vi "multiply value.vi"(6 "label":T1, 8 "error in (no error)":errorcluster, 10 "B":refnum<class "Value.lvclass">, 11 "A":refnum<class "Value.lvclass">) -> (0 "error out":errorcluster, 2 "C":refnum<class "Value.lvclass">, 3 "A out":refnum<class "Value.lvclass">)   [LabVIEW 2023, in "LabGRAD.lvlib" / "Value.lvclass"]
uses:
  Value.lvclass
  UiObjects/string control.ctl
  operation.ctl
  Value.lvclass/Value.ctl
  UiObjects/UiObjects.lvclass
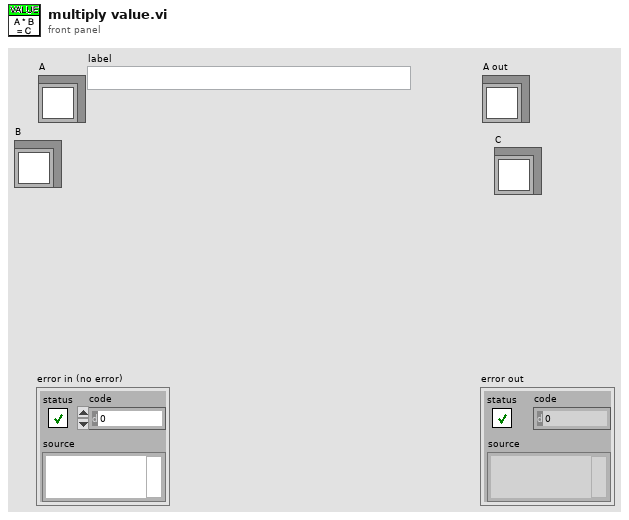
[diagram p1: front panel]
types:
  T1 = typedef "UiObjects.lvlib/UiObjects.lvclass/string control.ctl" = string
  T2 = typedef "LabGRAD.lvlib/Value.lvclass/operation.ctl" = enum16{"nop", "add", "subtract", "power", "multiply", "divide"}
  T3 = typedef "UiObjects.lvlib/UiObjects.lvclass/numeric value control.ctl" = dbl
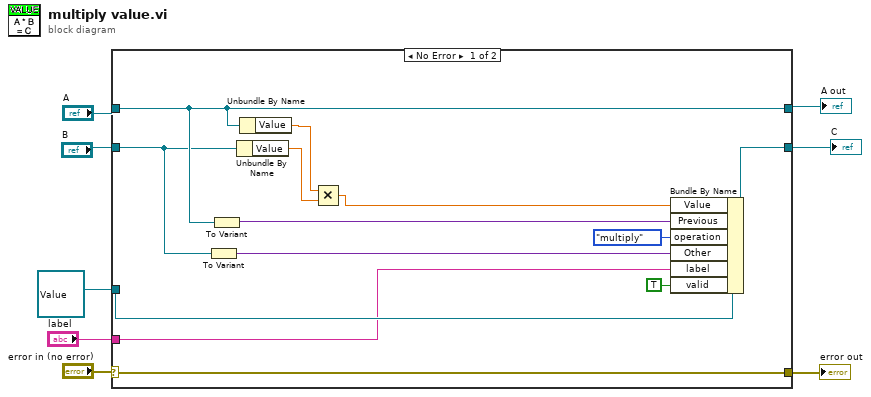
[diagram p0: block diagram]
diagram:
  n1 = case shown="No Error" "error in (no error)" {
    selector: "error in (no error)" -> [w21 w24]
    tunnel: [w21 w24] -> w5
    tunnel: [w18 w23] -> w6
    tunnel: "A" -> [w18 w23]
    tunnel: "B" -> [w17 _]
    tunnel: [w16 w22] -> w2
    tunnel: refnum<class "Value.lvclass"> refnum ("B") -> [w14 w22]
    tunnel: "label" -> [w10 _]
    frame No Error {
      n2 = To Variant(anything=w17) -> (Variant=w12:variant)
      n3 = To Variant(anything=w18) -> (Variant=w11:variant)
      n4 = Unbundle By Name(w17) -> ("Value"=w19:T3)
      n5 = Unbundle By Name(w18) -> ("Value"=w20:T3)
      n6 = Multiply(x=w20, y=w19) -> (x*y=w15:T3)
      n7 = Bundle By Name(cluster=w14, "Value"=w15, "Previous"=w11, "operation"=operation."multiply", "Other"=w12, "label"=w10, "valid"=TRUE) -> (w16:refnum<class "Value.lvclass">)
    }
    frame Error {
    }
  }
  "error out" <- w5
  "A out" <- w6
  "C" <- w2
